vi "caseselector.vi"() -> ()   [LabVIEW 2020]
panel:
  in  "milliseconds to wait":u32
  in  "button name (\"OK\")":string
  in  "message":string
  out "Numeric":dbl
  out "italy temp 2":dbl=25.348837209302324
  in  "Numeric 2":dbl
  out "italy temp":dbl(slide) scale=0.0..2500.0
  in  "india temp":dbl(slide) scale=0.0..50.0
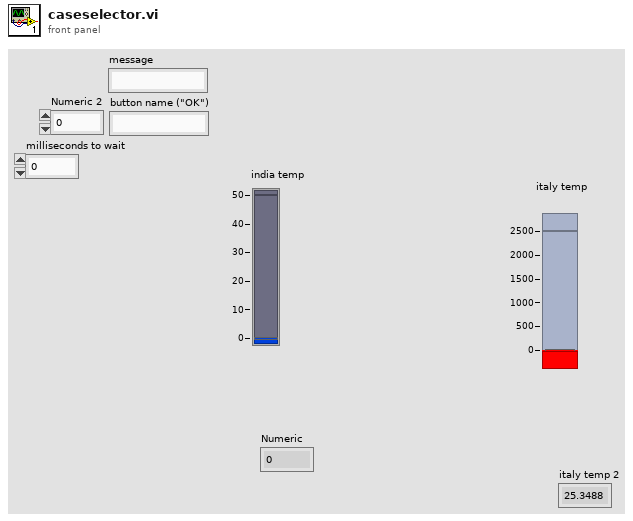
[diagram p1: front panel]
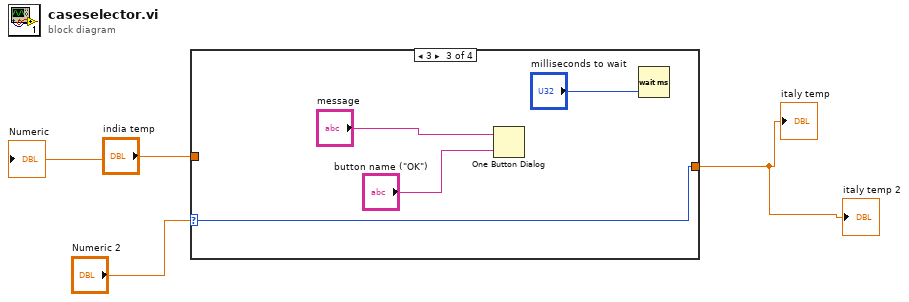
[diagram p0: block diagram]
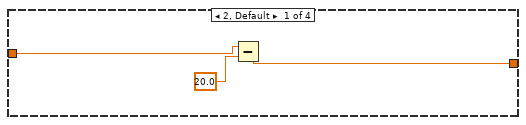
[diagram p2: hidden frame]
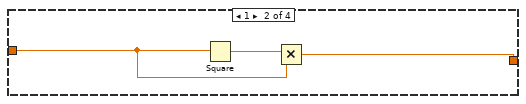
[diagram p3: hidden frame]
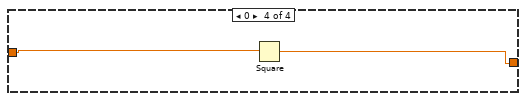
[diagram p4: hidden frame]
diagram:
  n1 = case shown="3" "Numeric 2" {
    selector: "Numeric 2" -> [_ _ w13 _]
    tunnel: [w4 w7 w13 w15] -> w2
    tunnel: "india temp" -> [w6 w8 _ w14]
    frame 2, Default {
      n2 = Subtract(x=w6, y=20.0) -> (x-y=w4:dbl)
    }
    frame 1 {
      n3 = Square(x=w8) -> (x^2=w9:dbl)
      n4 = Multiply(x=w9, y=w8) -> (x*y=w7:dbl)
    }
    frame 3 {
      n5 = One Button Dialog(message="message", button name ("OK")="button name (\"OK\")") -> ()  [unwired: 1 out]
      n6 = Wait (ms)(milliseconds to wait="milliseconds to wait") -> ()  [unwired: 1 out]
    }
    frame 0 {
      n7 = Square(x=w14) -> (x^2=w15:dbl)
    }
  }
  "italy temp" <- w2
  "italy temp 2" <- w2
  "Numeric" <- "india temp"
